vi "Lab Panel V5.24.vi"() -> ()   [LabVIEW 2013] (continued)
                    n2903 = Number To Fractional String(number=w5323, precision (6)=w5281) -> (F-format string=w5321:string)  [unwired: 2 in]
                    n2904 = Number To Fractional String(number=w5333, precision (6)=w5281) -> (F-format string=w5331:string)  [unwired: 2 in]
                    n2905 = Number To Fractional String(number=w5328, precision (6)=w5281) -> (F-format string=w5326:string)  [unwired: 2 in]
                    n2906 = Number To Fractional String(number=w5313, precision (6)=w5281) -> (F-format string=w5311:string)  [unwired: 2 in]
                    n2907 = Number To Fractional String(number=w5318, precision (6)=w5281) -> (F-format string=w5316:string)  [unwired: 2 in]
                    n2908 = Number To Fractional String(number=w5343, precision (6)=w5281) -> (F-format string=w5341:string)  [unwired: 2 in]
                    n2909 = Number To Fractional String(number=w5308, precision (6)=w5281) -> (F-format string=w5306:string)  [unwired: 2 in]
                    n2910 = Number To Fractional String(number=w5348, precision (6)=w5281) -> (F-format string=w5346:string)  [unwired: 2 in]
                    n2911 = Number To Fractional String(number=w5350, precision (6)=w5281) -> (F-format string=w5303:string)  [unwired: 2 in]
                    n2912 = Concatenate Strings(w5280, w5322, w5280, w5321, w5280, w5320) -> (w5296:string)
                    n2913 = Concatenate Strings(w5280, w5317, w5280, w5316, w5280, w5315) -> (w5295:string)
                    n2914 = Concatenate Strings(w5280, w5312, w5280, w5311, w5280, w5310) -> (w5294:string)
                    n2915 = Concatenate Strings(w5280, w5307, w5280, w5306, w5280, w5305) -> (w5293:string)
                    n2916 = Concatenate Strings(w5280, w5304, w5280, w5303, w5280, w5302) -> (w5292:string)
                    n2917 = Concatenate Strings(w5280, w5347, w5280, w5346, w5280, w5345) -> (w5301:string)
                    n2918 = Concatenate Strings(w5280, w5327, w5280, w5326, w5280, w5325) -> (w5297:string)
                    n2919 = Concatenate Strings(w5280, w5342, w5280, w5341, w5280, w5340) -> (w5300:string)
                    n2920 = Concatenate Strings(w5280, w5339, w5280, w5338, w5280, w5335) -> (w5299:string)
                    n2921 = Concatenate Strings(w5280, w5332, w5280, w5331, w5280, w5330) -> (w5298:string)
                    n2922 = Concatenate Strings("]", "\r") -> (w5277:string)
                    n2923 = Concatenate Strings(w5272, w5297, w5277) -> (w5287:string)
                    n2924 = Concatenate Strings(w5274, w5299, w5277) -> (w5289:string)
                    n2925 = Concatenate Strings(w5273, w5298, w5277) -> (w5288:string)
                    n2926 = Concatenate Strings(w5269, w5294, w5277) -> (w5284:string)
                    n2927 = Concatenate Strings(w5270, w5293, w5277) -> (w5285:string)
                    n2928 = Concatenate Strings(w5268, w5295, w5277) -> (w5283:string)
                    n2929 = Concatenate Strings(w5267, w5296, w5277) -> (w5282:string)
                    n2930 = Concatenate Strings(w5271, w5292, w5277) -> (w5286:string)
                    n2931 = Concatenate Strings(w5275, w5300, w5277) -> (w5290:string)
                    n2932 = Concatenate Strings(w5276, w5301, w5277) -> (w5291:string)
                    n2933 = Concatenate Strings(w5291, w5290, w5289, w5288, w5287, w5282, w5283, w5284, w5285, w5286) -> (w5260:string)
                    n2934 = Concatenate Strings("[PANEL/", "DESC/", "CYCLES/", "MINS/", "STATUS]", "\r", w5260) -> (w5259:string)
                    "MAIL REPORT" <- w5259
                    n2935 = global write "Global display 3.vi" "log all"(w5259) -> ()
                  }
                  frame #2 {
                    w5390 = "END"
                    n2936 = local read "mail control"() -> (w5391:string)
                    n2937 = case shown="False" w5386 {
                      tunnel: w5391 -> [w5415 _]
                      tunnel: w5390 -> [w5414 _]
                      tunnel: [w5413 FALSE] -> w5376
                      frame False {
                        n2938 = Equal?(x=w5415, y=w5414) -> (x = y?=w5413:bool)
                      }
                      frame True {
                      }
                    }
                    n2939 = case shown="False" w5392 {
                      tunnel: w5391 -> [w5431 _]
                      tunnel: w5390 -> [w5430 _]
                      tunnel: [w5429 FALSE] -> w5380
                      frame False {
                        n2940 = Equal?(x=w5431, y=w5430) -> (x = y?=w5429:bool)
                      }
                      frame True {
                      }
                    }
                    n2941 = case shown="False" w5389 {
                      tunnel: w5391 -> [w5427 _]
                      tunnel: w5390 -> [w5426 _]
                      tunnel: [w5425 FALSE] -> w5379
                      frame False {
                        n2942 = Equal?(x=w5427, y=w5426) -> (x = y?=w5425:bool)
                      }
                      frame True {
                      }
                    }
                    n2943 = case shown="False" w5387 {
                      tunnel: w5391 -> [w5419 _]
                      tunnel: w5390 -> [w5418 _]
                      tunnel: [w5417 FALSE] -> w5377
                      frame False {
                        n2944 = Equal?(x=w5419, y=w5418) -> (x = y?=w5417:bool)
                      }
                      frame True {
                      }
                    }
                    n2945 = case shown="False" w5388 {
                      tunnel: w5391 -> [w5423 _]
                      tunnel: w5390 -> [w5422 _]
                      tunnel: [w5421 FALSE] -> w5378
                      frame False {
                        n2946 = Equal?(x=w5423, y=w5422) -> (x = y?=w5421:bool)
                      }
                      frame True {
                      }
                    }
                    n2947 = Or(x=w5378, y=w5377) -> (x .or. y?=w5369:bool)
                    n2948 = Or(x=w5380, y=w5379) -> (x .or. y?=w5370:bool)
                    n2949 = Or(x=w5370, y=w5369) -> (x .or. y?=w5365:bool)
                    n2950 = case shown="False" w5382 {
                      tunnel: w5391 -> [w5399 _]
                      tunnel: w5390 -> [w5398 _]
                      tunnel: [w5397 FALSE] -> w5371
                      frame False {
                        n2951 = Equal?(x=w5399, y=w5398) -> (x = y?=w5397:bool)
                      }
                      frame True {
                      }
                    }
                    n2952 = case shown="False" w5381 {
                      tunnel: w5391 -> [w5395 _]
                      tunnel: w5390 -> [w5394 _]
                      tunnel: [w5393 FALSE] -> w5375
                      frame False {
                        n2953 = Equal?(x=w5395, y=w5394) -> (x = y?=w5393:bool)
                      }
                      frame True {
                      }
                    }
                    n2954 = case shown="False" w5383 {
                      tunnel: w5391 -> [w5403 _]
                      tunnel: w5390 -> [w5402 _]
                      tunnel: [w5401 FALSE] -> w5372
                      frame False {
                        n2955 = Equal?(x=w5403, y=w5402) -> (x = y?=w5401:bool)
                      }
                      frame True {
                      }
                    }
                    n2956 = case shown="False" w5385 {
                      tunnel: w5391 -> [w5411 _]
                      tunnel: w5390 -> [w5410 _]
                      tunnel: [w5409 FALSE] -> w5374
                      frame False {
                        n2957 = Equal?(x=w5411, y=w5410) -> (x = y?=w5409:bool)
                      }
                      frame True {
                      }
                    }
                    n2958 = case shown="False" w5384 {
                      tunnel: w5391 -> [w5407 _]
                      tunnel: w5390 -> [w5406 _]
                      tunnel: [w5405 FALSE] -> w5373
                      frame False {
                        n2959 = Equal?(x=w5407, y=w5406) -> (x = y?=w5405:bool)
                      }
                      frame True {
                      }
                    }
                    n2960 = Or(x=w5374, y=w5373) -> (x .or. y?=w5368:bool)
                    n2961 = Or(x=w5372, y=w5371) -> (x .or. y?=w5367:bool)
                    n2962 = Or(x=w5375, y=w5376) -> (x .or. y?=w5363:bool)
                    n2963 = Or(x=w5368, y=w5367) -> (x .or. y?=w5366:bool)
                    n2964 = Or(x=w5365, y=w5366) -> (x .or. y?=w5364:bool)
                    n2965 = Or(x=w5364, y=w5363) -> (x .or. y?=w5362:bool)
                  }
                  frame #3 {
                    n2966 = local read "on loops"() -> (w5445:dbl)
                    n2967 = local read "jig cycle"() -> (w5442:dbl)
                    n2968 = local read "Send Mail Now"() -> (w5436:bool)
                    n2969 = Add(x=w5445, y=3.0) -> (x+y=w5443:dbl)
                    n2970 = Equal?(x=w5442, y=w5443) -> (x = y?=w5437:bool)
                    n2971 = And(x=w5437, y=w5436) -> (x .and. y?=w5435:bool)
                    n2972 = And(x=w5441, y=w5437) -> (x .and. y?=w5440:bool)
                    n2973 = And(x=w5440, y=w5439) -> (x .and. y?=w5438:bool)
                    n2974 = Or(x=w5438, y=w5435) -> (x .or. y?=w5434:bool)
                    n2975 = case shown="True" w5434 {
                      tunnel: w5450 -> [_ w5456]
                      tunnel: w5449 -> [_ w5455]
                      tunnel: "Lab Panel Test Status" -> [_ w5454]
                      tunnel: w5447 -> [_ w5453]
                      tunnel: w5446 -> [_ w5452]
                      tunnel: w5433 -> [_ w5451]
                      frame False {
                      }
                      frame True {
                        n2976 = stacked-sequence {
                          tunnel: w5456 -> [w5464 _]
                          tunnel: w5455 -> [w5463 _]
                          tunnel: w5454 -> [w5462 _]
                          tunnel: w5453 -> [w5461 _]
                          tunnel: w5452 -> [w5460 _]
                          tunnel: w5451 -> [w5459 _]
                          frame #0 {
                            n2977 = call "sub vi - send mail v5.vi"("TO:"=w5464, "subject"=w5462, "from"=w5460, "out going server"=w5461, "message"=w5463) -> ("error out"=w5458:errorcluster)  [unwired: 10 in]
                            n2978 = Bundle(cluster=w5459, "mail error"=w5458) -> (w5457:T7)  [unwired: 6 in]
                            n2979 = local write "MAIL SETTINGS"(w5457) -> ()
                          }
                          frame #1 {
                            n2980 = local write "mail control"("") -> ()
                            n2981 = local write "Send Mail Now"(FALSE) -> ()
                          }
                        }
                      }
                    }
                  }
                }
              }
            }
          }
          frame #19 {
            # "save jig cycle values once all run switches are off"
            n2982 = stacked-sequence {
              tunnel: w5476 -> [_ w5505]
              tunnel: w5475 -> [_ w5504]
              tunnel: w5474 -> [_ w5503]
              tunnel: w5473 -> [_ w5502]
              tunnel: w5472 -> [_ w5501]
              tunnel: w5471 -> [_ w5500]
              tunnel: w5470 -> [_ w5499]
              tunnel: w5469 -> [_ w5498]
              tunnel: w5468 -> [_ w5497]
              tunnel: w5467 -> [_ w5496]
              frame #0 {
              }
              frame #1 {
                n2983 = Not(x=w5496) -> (.not. x?=w5479:bool)
                n2984 = Not(x=w5504) -> (.not. x?=w5494:bool)
                n2985 = Not(x=w5501) -> (.not. x?=w5489:bool)
                n2986 = Not(x=w5499) -> (.not. x?=w5485:bool)
                n2987 = Not(x=w5497) -> (.not. x?=w5481:bool)
                n2988 = Not(x=w5505) -> (.not. x?=w5495:bool)
                n2989 = Not(x=w5503) -> (.not. x?=w5493:bool)
                n2990 = Not(x=w5500) -> (.not. x?=w5487:bool)
                n2991 = Not(x=w5502) -> (.not. x?=w5491:bool)
                n2992 = Not(x=w5498) -> (.not. x?=w5483:bool)
                n2993 = local read "Save JC"() -> (w5507:bool)
                n2994 = And(x=w5495, y=w5494) -> (x .and. y?=w5492:bool)
                n2995 = And(x=w5492, y=w5493) -> (x .and. y?=w5490:bool)
                n2996 = And(x=w5490, y=w5491) -> (x .and. y?=w5488:bool)
                n2997 = And(x=w5488, y=w5489) -> (x .and. y?=w5486:bool)
                n2998 = And(x=w5486, y=w5487) -> (x .and. y?=w5484:bool)
                n2999 = And(x=w5484, y=w5485) -> (x .and. y?=w5482:bool)
                n3000 = And(x=w5482, y=w5483) -> (x .and. y?=w5480:bool)
                n3001 = And(x=w5480, y=w5481) -> (x .and. y?=w5478:bool)
                n3002 = And(x=w5478, y=w5479) -> (x .and. y?=w5477:bool)
                n3003 = And(x=w5477, y=w5507) -> (x .and. y?=w5506:bool)
                n3004 = case shown="True" w5506 {
                  tunnel: w5477 -> [w5508 _]
                  frame False {
                    n3005 = case shown="False" w5508 {
                      frame False {
                        n3006 = local write "Save JC"(TRUE) -> ()
                      }
                      frame True {
                      }
                    }
                  }
                  frame True {
                    n3007 = stacked-sequence {
                      frame #0 {
                        n3008 = String To Path(string="c:\\crabtree\\Jig Cycles\\") -> (path=w5520:path)
                        n3009 = Build Path(base path=w5520, name or relative path="jigcycles.bin") -> (appended path=w5518:path)
                        n3010 = Create Folder(path (use dialog)=w5520) -> (error out=w5522:errorcluster)  [unwired: 2 in, 2 out]
                        n3011 = local read "JIG RELAY CYCLES"() -> (w5512:T8)
                        n3012 = call <vilib>:"Clear Errors.vi"("error in (no error)"=w5522) -> ()  [unwired: 6 in, 1 out]
                        n3013 = local write "Save JC"(FALSE) -> ()
                        n3014 = Open/Create/Replace File(file path (use dialog)=w5518, operation (0:open)=T17."replace or create") -> (refnum out=w5516:refnum<file>, error out=w5517:errorcluster)  [unwired: 4 in, 1 out]
                        n3015 = Write to Binary File(file (use dialog)=w5516, data=w5512, error in=w5517) -> (refnum out=w5515:refnum<file>, error out=w5514:errorcluster)  [unwired: 3 in, 1 out]
                        n3016 = Close File(refnum=w5515, error in=w5514) -> (error out=w5513:errorcluster)  [unwired: 1 out]
                        n3017 = local write "data file error"(w5513) -> ()
                      }
                      frame #1 {
                        n3018 = local read "JIG RELAY CYCLES"() -> (w5545:T8)
                        n3019 = Unbundle By Name(w5545) -> ("LAB01-1"=w5540:dbl, "LAB01-2"=w5539:dbl, "LAB02-1"=w5537:dbl, "LAB02-2"=w5536:dbl, "LAB03-1"=w5534:dbl, "LAB03-2"=w5531:dbl, "LAB04-1"=w5530:dbl, "LAB04-2"=w5528:dbl, "LAB05-1"=w5526:dbl, "LAB05-2"=w5524:dbl)
                        n3020 = stacked-sequence {
                          tunnel: w5540 -> [w5548 _ _ _ _ _ _ _ _ _]
                          tunnel: 1000000 -> [w5551 w5561 w5571 w5581 w5591 w5601 w5611 w5621 w5631 w5641]
                          tunnel: [w5549 _ _ _ _ _ _ _ _ _] -> w5543
                          tunnel: "TEST STATION HAS REACHED 1 MILLION CYCLES, REPLACE  CONTROL RELAYS" -> [w5547 w5559 w5569 w5579 w5589 w5599 w5609 w5619 w5629 w5639]
                          tunnel: [_ w5558 _ _ _ _ _ _ _ _] -> w5541
                          tunnel: w5539 -> [_ w5557 _ _ _ _ _ _ _ _]
                          tunnel: [_ _ w5568 _ _ _ _ _ _ _] -> w5538
                          tunnel: w5537 -> [_ _ w5567 _ _ _ _ _ _ _]
                          tunnel: w5536 -> [_ _ _ w5578 _ _ _ _ _ _]
                          tunnel: [_ _ _ w5577 _ _ _ _ _ _] -> w5535
                          tunnel: w5534 -> [_ _ _ _ w5588 _ _ _ _ _]
                          tunnel: [_ _ _ _ w5587 _ _ _ _ _] -> w5533
                          tunnel: [_ _ _ _ _ w5598 _ _ _ _] -> w5532
                          tunnel: w5531 -> [_ _ _ _ _ w5597 _ _ _ _]
                          tunnel: w5530 -> [_ _ _ _ _ _ w5608 _ _ _]
                          tunnel: [_ _ _ _ _ _ w5607 _ _ _] -> w5529
                          tunnel: w5528 -> [_ _ _ _ _ _ _ w5618 _ _]
                          tunnel: [_ _ _ _ _ _ _ w5617 _ _] -> w5527
                          tunnel: w5526 -> [_ _ _ _ _ _ _ _ w5628 _]
                          tunnel: [_ _ _ _ _ _ _ _ w5627 _] -> w5525
                          tunnel: w5524 -> [_ _ _ _ _ _ _ _ _ w5638]
                          tunnel: [_ _ _ _ _ _ _ _ _ w5637] -> w5523
                          frame #0 {
                            n3021 = Greater?(x=w5548, y=w5551) -> (0:w5550:bool)
                            n3022 = case shown="True" w5550 {
                              tunnel: [w5552 0] -> w5549
                              tunnel: w5548 -> [w5552 _]
                              tunnel: w5547 -> [_ w5553]
                              frame False {
                              }
                              frame True {
                                n3023 = Concatenate Strings("LA01-1 ", w5553) -> (w5556:string)
                                n3024 = One Button Dialog(message=w5556) -> ()  [unwired: 1 in, 1 out]
                              }
                            }
                          }
                          frame #1 {
                            n3025 = Greater?(x=w5557, y=w5561) -> (0:w5560:bool)
                            n3026 = case shown="True" w5560 {
                              tunnel: [w5562 0] -> w5558
                              tunnel: w5557 -> [w5562 _]
                              tunnel: w5559 -> [_ w5563]
                              frame False {
                              }
                              frame True {
                                n3027 = Concatenate Strings("LA01-2 ", w5563) -> (w5566:string)
                                n3028 = One Button Dialog(message=w5566) -> ()  [unwired: 1 in, 1 out]
                              }
                            }
                          }
                          frame #2 {
                            n3029 = Greater?(x=w5567, y=w5571) -> (0:w5570:bool)
                            n3030 = case shown="True" w5570 {
                              tunnel: [w5572 0] -> w5568
                              tunnel: w5567 -> [w5572 _]
                              tunnel: w5569 -> [_ w5573]
                              frame False {
                              }
                              frame True {
                                n3031 = Concatenate Strings("LA02-1 ", w5573) -> (w5576:string)
                                n3032 = One Button Dialog(message=w5576) -> ()  [unwired: 1 in, 1 out]
                              }
                            }
                          }
                          frame #3 {
                            n3033 = Greater?(x=w5578, y=w5581) -> (0:w5580:bool)
                            n3034 = case shown="True" w5580 {
                              tunnel: [w5582 0] -> w5577
                              tunnel: w5578 -> [w5582 _]
                              tunnel: w5579 -> [_ w5583]
                              frame False {
                              }
                              frame True {
                                n3035 = Concatenate Strings("LA02-2 ", w5583) -> (w5586:string)
                                n3036 = One Button Dialog(message=w5586) -> ()  [unwired: 1 in, 1 out]
                              }
                            }
                          }
                          frame #4 {
                            n3037 = Greater?(x=w5588, y=w5591) -> (0:w5590:bool)
                            n3038 = case shown="True" w5590 {
                              tunnel: [w5592 0] -> w5587
                              tunnel: w5588 -> [w5592 _]
                              tunnel: w5589 -> [_ w5593]
                              frame False {
                              }
                              frame True {
                                n3039 = Concatenate Strings("LA03-1 ", w5593) -> (w5596:string)
                                n3040 = One Button Dialog(message=w5596) -> ()  [unwired: 1 in, 1 out]
                              }
                            }
                          }
                          frame #5 {
                            n3041 = Greater?(x=w5597, y=w5601) -> (0:w5600:bool)
                            n3042 = case shown="True" w5600 {
                              tunnel: [w5602 0] -> w5598
                              tunnel: w5597 -> [w5602 _]
                              tunnel: w5599 -> [_ w5603]
                              frame False {
                              }
                              frame True {
                                n3043 = Concatenate Strings("LA03-2 ", w5603) -> (w5606:string)
                                n3044 = One Button Dialog(message=w5606) -> ()  [unwired: 1 in, 1 out]
                              }
                            }
                          }
                          frame #6 {
                            n3045 = Greater?(x=w5608, y=w5611) -> (0:w5610:bool)
                            n3046 = case shown="True" w5610 {
                              tunnel: [w5612 0] -> w5607
                              tunnel: w5608 -> [w5612 _]
                              tunnel: w5609 -> [_ w5613]
                              frame False {
                              }
                              frame True {
                                n3047 = Concatenate Strings("LA04-1 ", w5613) -> (w5616:string)
                                n3048 = One Button Dialog(message=w5616) -> ()  [unwired: 1 in, 1 out]
                              }
                            }
                          }
                          frame #7 {
                            n3049 = Greater?(x=w5618, y=w5621) -> (0:w5620:bool)
                            n3050 = case shown="True" w5620 {
                              tunnel: [w5622 0] -> w5617
                              tunnel: w5618 -> [w5622 _]
                              tunnel: w5619 -> [_ w5623]
                              frame False {
                              }
                              frame True {
                                n3051 = Concatenate Strings("LA04-2 ", w5623) -> (w5626:string)
                                n3052 = One Button Dialog(message=w5626) -> ()  [unwired: 1 in, 1 out]
                              }
                            }
                          }
                          frame #8 {
                            n3053 = Greater?(x=w5628, y=w5631) -> (0:w5630:bool)
                            n3054 = case shown="True" w5630 {
                              tunnel: [w5632 0] -> w5627
                              tunnel: w5628 -> [w5632 _]
                              tunnel: w5629 -> [_ w5633]
                              frame False {
                              }
                              frame True {
                                n3055 = Concatenate Strings("LA05-1 ", w5633) -> (w5636:string)
                                n3056 = One Button Dialog(message=w5636) -> ()  [unwired: 1 in, 1 out]
                              }
                            }
                          }
                          frame #9 {
                            n3057 = Greater?(x=w5638, y=w5641) -> (0:w5640:bool)
                            n3058 = case shown="True" w5640 {
                              tunnel: [w5642 0] -> w5637
                              tunnel: w5638 -> [w5642 _]
                              tunnel: w5639 -> [_ w5643]
                              frame False {
                              }
                              frame True {
                                n3059 = Concatenate Strings("LA05-2 ", w5643) -> (w5646:string)
                                n3060 = One Button Dialog(message=w5646) -> ()  [unwired: 1 in, 1 out]
                              }
                            }
                          }
                        }
                        n3061 = Bundle By Name(cluster=w5545, "LAB01-1"=w5543, "LAB01-2"=w5541, "LAB02-1"=w5538, "LAB02-2"=w5535, "LAB03-1"=w5533, "LAB03-2"=w5532, "LAB04-1"=w5529, "LAB04-2"=w5527, "LAB05-1"=w5525, "LAB05-2"=w5523) -> (w5544:T8)
                        n3062 = local write "JIG RELAY CYCLES"(w5544) -> ()
                      }
                    }
                  }
                }
              }
            }
          }
          frame #20 {
            # "get temperature values"
            n3063 = local read "Simulate"() -> (w5659:bool)
            n3064 = local read "Temp Test Cal"() -> (w5656:dbl)
            n3065 = stacked-sequence {
              seq-local: [w5661 _] -> [_ w5706]
              tunnel: w5659 -> [_ w5719]
              tunnel: T14 {"1  (A) cal"=1.0, "1 (V) cal"=1.0, "1 (PF) cal"=1.0, "1 (TL) cal"=1.0, "1 (TN) cal"=1.0, "2 (A) cal"=1.0, "2 (V) cal"=1.0, "2 (PF) cal"=1.0, "2 (TL) cal"=1.0, "2 (TN) cal"=1.0} ("CAL LAB01") -> [_ w5718]
              tunnel: w5657 -> [_ w5717]
              tunnel: w5656 -> [_ w5716]
              tunnel: w5655 -> [_ w5715]
              tunnel: w5654 -> [_ w5714]
              tunnel: w5653 -> [_ w5713]
              tunnel: w5652 -> [_ w5712]
              tunnel: w5651 -> [_ w5711]
              tunnel: w5650 -> [_ w5710]
              tunnel: w5649 -> [_ w5709]
              tunnel: w5648 -> [_ w5708]
              tunnel: w5647 -> [_ w5707]
              frame #0 {
                # "only get temperature from initial valid temperature circuits"
                n3066 = local read "Select COM port"() -> (w5669:refnum<visa-resource-name>)
                "COM port" <- w5669
                n3067 = global write "Global 1.vi" "COM port"(w5669) -> ()
                n3068 = global write "Global 1.vi" "tmp dly lps"("Temp Delay Lps") -> ()
                n3069 = local read "Temp read loop"() -> (w5666:dbl)
                n3070 = global write "Global 1.vi" "dly value"("Temp Value") -> ()
                n3071 = local read "jig cycle"() -> (w5670:dbl)
                n3072 = local read "on loops"() -> (w5672:dbl)
                n3073 = Equal?(x=w5666, y=1) -> (x = y?=w5663:bool)
                n3074 = Add(x=w5672, y=3) -> (x+y=w5673:dbl)
                n3075 = Equal?(x=w5670, y=w5673) -> (x = y?=w5664:bool)
                n3076 = And(x=w5664, y=w5663) -> (x .and. y?=w5662:bool)
                n3077 = Or(x=w5662, y="Read Temp") -> (x .or. y?=w5661:bool)
                n3078 = case shown="True" w5661 {
                  frame False {
                  }
                  frame True {
                    n3079 = local read "Simulate"() -> (w5675:bool)
                    n3080 = local write "TEMP"(TRUE) -> ()
                    n3081 = local write "Read Temp"(FALSE) -> ()
                    n3082 = stacked-sequence {
                      tunnel: 1.0 -> [_ _ _ _ w5705]
                      tunnel: w5675 -> [_ _ _ _ w5704]
                      frame #0 {
                        # "only switch relay on to reset temp circuits if busy testing"
                        n3083 = local read "USB OUT 0"() -> (w5679:bool[])
                        n3084 = local read "USB OUT 2"() -> (w5681:bool[])
                        n3085 = local read "USB OUT 1"() -> (w5680:bool[])
                        n3086 = local read "Any Test Running"() -> (w5678:bool)
                        n3087 = Insert Into Array(array=w5681, index=7, new element=w5678) -> (w5682:bool[])
                        n3088 = call "sub vi - Drive Relays All v6.vi"("Array #2"=w5682, "Array #1"=w5680, "Array #0"=w5679) -> ()  [unwired: 8 in, 1 out]
                      }
                      frame #1 {
                        # "time delay"
                        n3089 = Wait (ms)(milliseconds to wait=500) -> ()  [unwired: 1 out]
                      }
                      frame #2 {
                        # "switch relay off"
                        n3090 = local read "USB OUT 0"() -> (w5685:bool[])
                        n3091 = local read "USB OUT 2"() -> (w5687:bool[])
                        n3092 = local read "USB OUT 1"() -> (w5686:bool[])
                        n3093 = Insert Into Array(array=w5687, index=7, new element=FALSE) -> (w5688:bool[])
                        n3094 = call "sub vi - Drive Relays All v6.vi"("Array #2"=w5688, "Array #1"=w5686, "Array #0"=w5685) -> ()  [unwired: 8 in, 1 out]
                      }
                      frame #3 {
                        # "time delay"
                        n3095 = Wait (ms)(milliseconds to wait=200) -> ()  [unwired: 1 out]
                      }
                      frame #4 {
                        # "read all valid temp circuits"
                        n3096 = local read "LAB01-TP"() -> (w5697:bool)
                        n3097 = local read "LAB03-TP"() -> (w5695:bool)
                        n3098 = local read "LAB02-TP"() -> (w5696:bool)
                        n3099 = local read "LAB04-TP"() -> (w5694:bool)
                        n3100 = local read "LAB05-TP"() -> (w5698:bool)
                        n3101 = call "sub vi - GET ALL TEMP v7.vi"("LA01-EN"=w5697, "simulate"=w5704, "LA02-EN"=w5696, "LA03-EN"=w5695, "LA04-EN"=w5694, "LA05-EN"=w5698, "Gen Cal Value"=w5705) -> ("LOOP TIME"=→"Read Time":dbl, "LA01 TEMP"=w5703:T25, "LA02 TEMP"=w5702:T25, "LA03 TEMP"=w5701:T25, "LA04 TEMP"=w5700:T25, "error"=→"Error Temp":bool, "LA05 TEMP"=w5699:T25)  [unwired: 1 in, 1 out]
                        n3102 = local write "LAB01 TEMP"(w5703) -> ()
                        n3103 = local write "LAB02 TEMP"(w5702) -> ()
                        n3104 = local write "LAB03 TEMP"(w5701) -> ()
                        n3105 = local write "LAB04 TEMP"(w5700) -> ()
                        n3106 = local write "LAB05 TEMP"(w5699) -> ()
                      }
                    }
                  }
                }
              }
              frame #1 {
                n3107 = case shown="True" w5706 {
                  tunnel: w5719 -> [_ w5732]
                  tunnel: w5718 -> [_ w5731]
                  tunnel: w5717 -> [_ w5730]
                  tunnel: w5716 -> [_ w5729]
                  tunnel: w5715 -> [_ w5728]
                  tunnel: w5714 -> [_ w5727]
                  tunnel: w5713 -> [_ w5726]
                  tunnel: w5712 -> [_ w5725]
                  tunnel: w5711 -> [_ w5724]
                  tunnel: w5710 -> [_ w5723]
                  tunnel: w5709 -> [_ w5722]
                  tunnel: w5708 -> [_ w5721]
                  tunnel: w5707 -> [_ w5720]
                  frame False {
                  }
                  frame True {
                    n3108 = stacked-sequence {
                      tunnel: w5732 -> [_ w5745 w5790 w5835 w5880 w5925]
                      tunnel: w5731 -> [_ w5744 w5789 w5834 w5879 w5924]
                      tunnel: w5730 -> [_ w5734 _ _ _ _]
                      tunnel: w5729 -> [_ w5739 w5788 w5833 w5878 w5923]
                      tunnel: w5728 -> [_ w5733 _ _ _ _]
                      tunnel: w5727 -> [_ _ w5779 _ _ _]
                      tunnel: w5726 -> [_ _ w5778 _ _ _]
                      tunnel: w5725 -> [_ _ _ w5824 _ _]
                      tunnel: w5724 -> [_ _ _ w5823 _ _]
                      tunnel: w5723 -> [_ _ _ _ w5869 _]
                      tunnel: w5722 -> [_ _ _ _ w5868 _]
                      tunnel: w5721 -> [_ _ _ _ _ w5914]
                      tunnel: w5720 -> [_ _ _ _ _ w5913]
                      frame #0 {
                      }
                      frame #1 {
                        n3109 = case shown="False" w5745 {
                          tunnel: [w5776 w5777] -> w5761
                          tunnel: w5744 -> [_ w5777]
                          frame False {
                            n3110 = local read "CAL LAB01"() -> (w5776:T14)
                          }
                          frame True {
                          }
                        }
                        n3111 = local read "TEMP LA01"() -> (w5752:T9)
                        n3112 = local read "LAB01 TEMP"() -> (w5751:T12)
                        n3113 = call "sub vi - temperature delay v3.vi"("2-run"=w5733, "1-run"=w5734, "temp values IN"=w5752, "temp signals"=w5751) -> ("T2-N"=w5747:dbl, "T2-L"=w5748:dbl, "T1-N"=w5749:dbl, "T1-L"=w5750:dbl, "temp values OUT"=w5746:T44)  [unwired: 3 in]
                        n3114 = Unbundle By Name(w5761) -> ("1 (TL) cal"=w5756:dbl, "1 (TN) cal"=w5755:dbl, "2 (TL) cal"=w5754:dbl, "2 (TN) cal"=w5753:dbl)  [unwired: 6 out]
                        n3115 = local write "TEMP LA01"(w5746) -> ()
                        n3116 = Multiply(x=w5750, y=w5756) -> (x*y=w5743:dbl)
                        n3117 = Multiply(x=w5749, y=w5755) -> (x*y=w5741:dbl)
                        n3118 = Multiply(x=w5748, y=w5754) -> (x*y=w5738:dbl)
                        n3119 = Multiply(x=w5747, y=w5753) -> (x*y=w5737:dbl)
                        n3120 = case shown="True" w5734 {
                          tunnel: w5743 -> [w5770 w5775]
                          tunnel: w5739 -> [_ w5773]
                          tunnel: [w5770 w5774] -> w5742
                          tunnel: w5741 -> [w5769 w5772]
                          tunnel: [w5769 w5771] -> w5740
                          frame False {
                          }
                          frame True {
                            n3121 = Multiply(x=w5773, y=w5772) -> (x*y=w5771:dbl)
                            n3122 = Multiply(x=w5773, y=w5775) -> (x*y=w5774:dbl)
                          }
                        }
                        n3123 = case shown="True" w5733 {
                          tunnel: w5738 -> [w5763 w5768]
                          tunnel: w5739 -> [_ w5766]
                          tunnel: [w5763 w5767] -> w5736
                          tunnel: w5737 -> [w5762 w5765]
                          tunnel: [w5762 w5764] -> w5735
                          frame False {
                          }
                          frame True {
                            n3124 = Multiply(x=w5766, y=w5765) -> (x*y=w5764:dbl)
                            n3125 = Multiply(x=w5766, y=w5768) -> (x*y=w5767:dbl)
                          }
                        }
                        n3126 = local read "SIG LAB01-2"() -> (w5758:T2)
                        n3127 = local read "SIG LAB01-1"() -> (w5760:T2)
                        n3128 = Bundle By Name(cluster=w5760, "Tmp Live"=w5742, "Tmp Neut"=w5740) -> (w5759:T2)
                        n3129 = Bundle By Name(cluster=w5758, "Tmp Live"=w5736, "Tmp Neut"=w5735) -> (w5757:T2)
                        n3130 = local write "SIG LAB01-1"(w5759) -> ()
                        n3131 = local write "SIG LAB01-2"(w5757) -> ()
                      }
                      frame #2 {
                        n3132 = case shown="True" w5790 {
                          tunnel: [w5821 w5822] -> w5806
                          tunnel: w5789 -> [_ w5822]
                          frame False {
                            n3133 = local read "CAL LAB02"() -> (w5821:T15)
                          }
                          frame True {
                          }
                        }
                        n3134 = local read "LAB02 TEMP"() -> (w5797:T12)
                        n3135 = local read "TEMP LA02"() -> (w5796:T9)
                        n3136 = call "sub vi - temperature delay v3.vi"("2-run"=w5778, "1-run"=w5779, "temp values IN"=w5796, "temp signals"=w5797) -> ("T2-N"=w5791:dbl, "T2-L"=w5792:dbl, "T1-N"=w5793:dbl, "T1-L"=w5794:dbl, "temp values OUT"=w5795:T44)  [unwired: 3 in]
                        n3137 = Unbundle By Name(w5806) -> ("1 (TL) cal"=w5801:dbl, "1 (TN) cal"=w5800:dbl, "2 (TL) cal"=w5799:dbl, "2 (TN) cal"=w5798:dbl)  [unwired: 6 out]
                        n3138 = local write "TEMP LA02"(w5795) -> ()
                        n3139 = Multiply(x=w5794, y=w5801) -> (x*y=w5787:dbl)
                        n3140 = Multiply(x=w5793, y=w5800) -> (x*y=w5786:dbl)
                        n3141 = Multiply(x=w5792, y=w5799) -> (x*y=w5783:dbl)
                        n3142 = Multiply(x=w5791, y=w5798) -> (x*y=w5782:dbl)
                        n3143 = case shown="True" w5779 {
                          tunnel: w5787 -> [w5815 w5820]
                          tunnel: w5788 -> [_ w5818]
                          tunnel: [w5815 w5819] -> w5785
                          tunnel: w5786 -> [w5814 w5817]
                          tunnel: [w5814 w5816] -> w5784
                          frame False {
                          }
                          frame True {
                            n3144 = Multiply(x=w5818, y=w5817) -> (x*y=w5816:dbl)
                            n3145 = Multiply(x=w5818, y=w5820) -> (x*y=w5819:dbl)
                          }
                        }
                        n3146 = case shown="True" w5778 {
                          tunnel: w5783 -> [w5808 w5813]
                          tunnel: w5788 -> [_ w5811]
                          tunnel: [w5808 w5812] -> w5781
                          tunnel: w5782 -> [w5807 w5810]
                          tunnel: [w5807 w5809] -> w5780
                          frame False {
                          }
                          frame True {
                            n3147 = Multiply(x=w5811, y=w5810) -> (x*y=w5809:dbl)
                            n3148 = Multiply(x=w5811, y=w5813) -> (x*y=w5812:dbl)
                          }
                        }
                        n3149 = local read "SIG LAB02-2"() -> (w5803:T2)
                        n3150 = local read "SIG LAB02-1"() -> (w5805:T2)
                        n3151 = Bundle By Name(cluster=w5805, "Tmp Live"=w5785, "Tmp Neut"=w5784) -> (w5804:T2)
                        n3152 = Bundle By Name(cluster=w5803, "Tmp Live"=w5781, "Tmp Neut"=w5780) -> (w5802:T2)
                        n3153 = local write "SIG LAB02-1"(w5804) -> ()
                        n3154 = local write "SIG LAB02-2"(w5802) -> ()
                      }
                      frame #3 {
                        n3155 = case shown="False" w5835 {
                          tunnel: [w5866 w5867] -> w5851
                          tunnel: w5834 -> [_ w5867]
                          frame False {
                            n3156 = local read "CAL LAB03"() -> (w5866:T14)
                          }
                          frame True {
                          }
                        }
                        n3157 = local read "TEMP LA03"() -> (w5841:T9)
                        n3158 = local read "LAB03 TEMP"() -> (w5842:T12)
                        n3159 = call "sub vi - temperature delay v3.vi"("2-run"=w5823, "1-run"=w5824, "temp values IN"=w5841, "temp signals"=w5842) -> ("T2-N"=w5836:dbl, "T2-L"=w5837:dbl, "T1-N"=w5838:dbl, "T1-L"=w5839:dbl, "temp values OUT"=w5840:T44)  [unwired: 3 in]
                        n3160 = Unbundle By Name(w5851) -> ("1 (TL) cal"=w5846:dbl, "1 (TN) cal"=w5845:dbl, "2 (TL) cal"=w5844:dbl, "2 (TN) cal"=w5843:dbl)  [unwired: 6 out]
                        n3161 = local write "TEMP LA03"(w5840) -> ()
                        n3162 = Multiply(x=w5839, y=w5846) -> (x*y=w5832:dbl)
                        n3163 = Multiply(x=w5838, y=w5845) -> (x*y=w5831:dbl)
                        n3164 = Multiply(x=w5837, y=w5844) -> (x*y=w5828:dbl)
                        n3165 = Multiply(x=w5836, y=w5843) -> (x*y=w5827:dbl)
                        n3166 = case shown="True" w5823 {
                          tunnel: w5828 -> [w5853 w5858]
                          tunnel: w5833 -> [_ w5856]
                          tunnel: [w5853 w5857] -> w5826
                          tunnel: w5827 -> [w5852 w5855]
                          tunnel: [w5852 w5854] -> w5825
                          frame False {
                          }
                          frame True {
                            n3167 = Multiply(x=w5856, y=w5855) -> (x*y=w5854:dbl)
                            n3168 = Multiply(x=w5856, y=w5858) -> (x*y=w5857:dbl)
                          }
                        }
                        n3169 = case shown="True" w5824 {
                          tunnel: w5832 -> [w5860 w5865]
                          tunnel: w5833 -> [_ w5863]
                          tunnel: [w5860 w5864] -> w5830
                          tunnel: w5831 -> [w5859 w5862]
                          tunnel: [w5859 w5861] -> w5829
                          frame False {
                          }
                          frame True {
                            n3170 = Multiply(x=w5863, y=w5862) -> (x*y=w5861:dbl)
                            n3171 = Multiply(x=w5863, y=w5865) -> (x*y=w5864:dbl)
                          }
                        }
                        n3172 = local read "SIG LAB03-2"() -> (w5848:T2)
                        n3173 = local read "SIG LAB03-1"() -> (w5850:T2)
                        n3174 = Bundle By Name(cluster=w5850, "Tmp Live"=w5830, "Tmp Neut"=w5829) -> (w5849:T2)
                        n3175 = Bundle By Name(cluster=w5848, "Tmp Live"=w5826, "Tmp Neut"=w5825) -> (w5847:T2)
                        n3176 = local write "SIG LAB03-1"(w5849) -> ()
                        n3177 = local write "SIG LAB03-2"(w5847) -> ()
                      }
                      frame #4 {
                        n3178 = case shown="False" w5880 {
                          tunnel: [w5911 w5912] -> w5896
                          tunnel: w5879 -> [_ w5912]
                          frame False {
                            n3179 = local read "CAL LAB04"() -> (w5911:T14)
                          }
                          frame True {
                          }
                        }
                        n3180 = local read "LAB04 TEMP"() -> (w5886:T12)
                        n3181 = local read "TEMP LA04"() -> (w5887:T9)
                        n3182 = call "sub vi - temperature delay v3.vi"("2-run"=w5868, "1-run"=w5869, "temp values IN"=w5887, "temp signals"=w5886) -> ("T2-N"=w5881:dbl, "T2-L"=w5882:dbl, "T1-N"=w5883:dbl, "T1-L"=w5884:dbl, "temp values OUT"=w5885:T44)  [unwired: 3 in]
                        n3183 = Unbundle By Name(w5896) -> ("1 (TL) cal"=w5891:dbl, "1 (TN) cal"=w5890:dbl, "2 (TL) cal"=w5889:dbl, "2 (TN) cal"=w5888:dbl)  [unwired: 6 out]
                        n3184 = local write "TEMP LA04"(w5885) -> ()
                        n3185 = Multiply(x=w5884, y=w5891) -> (x*y=w5877:dbl)
                        n3186 = Multiply(x=w5883, y=w5890) -> (x*y=w5876:dbl)
                        n3187 = Multiply(x=w5882, y=w5889) -> (x*y=w5873:dbl)
                        n3188 = Multiply(x=w5881, y=w5888) -> (x*y=w5872:dbl)
                        n3189 = case shown="True" w5868 {
                          tunnel: w5873 -> [w5898 w5903]
                          tunnel: w5878 -> [_ w5901]
                          tunnel: [w5898 w5902] -> w5871
                          tunnel: w5872 -> [w5897 w5900]
                          tunnel: [w5897 w5899] -> w5870
                          frame False {
                          }
                          frame True {
                            n3190 = Multiply(x=w5901, y=w5900) -> (x*y=w5899:dbl)
                            n3191 = Multiply(x=w5901, y=w5903) -> (x*y=w5902:dbl)
                          }
                        }
                        n3192 = case shown="True" w5869 {
                          tunnel: w5877 -> [w5905 w5910]
                          tunnel: w5878 -> [_ w5908]
                          tunnel: [w5905 w5909] -> w5875
                          tunnel: w5876 -> [w5904 w5907]
                          tunnel: [w5904 w5906] -> w5874
                          frame False {
                          }
                          frame True {
                            n3193 = Multiply(x=w5908, y=w5907) -> (x*y=w5906:dbl)
                            n3194 = Multiply(x=w5908, y=w5910) -> (x*y=w5909:dbl)
                          }
                        }
                        n3195 = local read "SIG LAB04-2"() -> (w5893:T2)
                        n3196 = local read "SIG LAB04-1"() -> (w5895:T2)
                        n3197 = Bundle By Name(cluster=w5895, "Tmp Live"=w5875, "Tmp Neut"=w5874) -> (w5894:T2)
                        n3198 = Bundle By Name(cluster=w5893, "Tmp Live"=w5871, "Tmp Neut"=w5870) -> (w5892:T2)
                        n3199 = local write "SIG LAB04-1"(w5894) -> ()
                        n3200 = local write "SIG LAB04-2"(w5892) -> ()
                      }
                      frame #5 {
                        n3201 = case shown="False" w5925 {
                          tunnel: [w5956 w5957] -> w5941
                          tunnel: w5924 -> [_ w5957]
                          frame False {
                            n3202 = local read "CAL LAB05"() -> (w5956:T14)
                          }
                          frame True {
                          }
                        }
                        n3203 = local read "LAB05 TEMP"() -> (w5931:T12)
                        n3204 = local read "TEMP LA05"() -> (w5932:T9)
                        n3205 = call "sub vi - temperature delay v3.vi"("2-run"=w5913, "1-run"=w5914, "temp values IN"=w5932, "temp signals"=w5931) -> ("T2-N"=w5927:dbl, "T2-L"=w5928:dbl, "T1-N"=w5929:dbl, "T1-L"=w5930:dbl, "temp values OUT"=w5926:T44)  [unwired: 3 in]
                        n3206 = local write "TEMP LA05"(w5926) -> ()
                        n3207 = Unbundle By Name(w5941) -> ("1 (TL) cal"=w5933:dbl, "1 (TN) cal"=w5936:dbl, "2 (TL) cal"=w5935:dbl, "2 (TN) cal"=w5934:dbl)  [unwired: 6 out]
                        n3208 = Multiply(x=w5930, y=w5933) -> (x*y=w5922:dbl)
                        n3209 = Multiply(x=w5929, y=w5936) -> (x*y=w5921:dbl)
                        n3210 = Multiply(x=w5928, y=w5935) -> (x*y=w5918:dbl)
                        n3211 = Multiply(x=w5927, y=w5934) -> (x*y=w5917:dbl)
                        n3212 = case shown="True" w5913 {
                          tunnel: w5918 -> [w5943 w5948]
                          tunnel: w5923 -> [_ w5946]
                          tunnel: [w5943 w5947] -> w5916
                          tunnel: w5917 -> [w5942 w5945]
                          tunnel: [w5942 w5944] -> w5915
                          frame False {
                          }
                          frame True {
                            n3213 = Multiply(x=w5946, y=w5945) -> (x*y=w5944:dbl)
                            n3214 = Multiply(x=w5946, y=w5948) -> (x*y=w5947:dbl)
                          }
                        }
                        n3215 = case shown="True" w5914 {
                          tunnel: w5922 -> [w5950 w5955]
                          tunnel: w5923 -> [_ w5953]
                          tunnel: [w5950 w5954] -> w5920
                          tunnel: w5921 -> [w5949 w5952]
                          tunnel: [w5949 w5951] -> w5919
                          frame False {
                          }
                          frame True {
                            n3216 = Multiply(x=w5953, y=w5952) -> (x*y=w5951:dbl)
                            n3217 = Multiply(x=w5953, y=w5955) -> (x*y=w5954:dbl)
                          }
                        }
                        n3218 = local read "SIG LAB05-1"() -> (w5940:T2)
                        n3219 = Bundle By Name(cluster=w5940, "Tmp Live"=w5920, "Tmp Neut"=w5919) -> (w5939:T2)
                        n3220 = local read "SIG LAB05-2"() -> (w5938:T2)
                        n3221 = Bundle By Name(cluster=w5938, "Tmp Live"=w5916, "Tmp Neut"=w5915) -> (w5937:T2)
                        n3222 = local write "SIG LAB05-1"(w5939) -> ()
                        n3223 = local write "SIG LAB05-2"(w5937) -> ()
                      }
                    }
                  }
                }
              }
            }
          }
          frame #21 {
            # "write data to display panel"
            n3224 = global write "Global display 1.vi" "TEST 5-2"(w5992) -> ()
            n3225 = global write "Global display 1.vi" "TEST 4-2"(w5994) -> ()
            n3226 = global write "Global display 1.vi" "TEST 1-2"(w6000) -> ()
            n3227 = global write "Global display 1.vi" "TEST 3-1"(w5997) -> ()
            n3228 = global write "Global display 1.vi" "TEST 5-1"(w5993) -> ()
            n3229 = global write "Global display 1.vi" "TEST 1-1"(w6001) -> ()
            n3230 = global write "Global display 1.vi" "TEST 3-2"(w5996) -> ()
            n3231 = global write "Global display 1.vi" "TEST 4-1"(w5995) -> ()
            n3232 = global write "Global display 1.vi" "TEST 2-2"(w5998) -> ()
            n3233 = global write "Global display 1.vi" "TEST 2-1"(w5999) -> ()
            n3234 = global read "Global display 3.vi" "log 1-1"() -> (→"LOG LAB01-1":string)
            n3235 = global read "Global display 3.vi" "log 3-1"() -> (→"LOG LAB03-1":string)
            n3236 = global read "Global display 3.vi" "log 1-2"() -> (→"LOG LAB01-2":string)
            n3237 = property on="Tab Control 2" class="TabCtl (strict)"() -> ("Pages"=w5991:refnum<vi>[])  [unwired: 2 in, 2 out]
